vi "Diagnostics Message Loop.vi"(8 "error in (no error)":errorcluster, 11 "Message Queues":T1) -> (0 "error out":errorcluster)   [LabVIEW 2021, in "Diagnostics.lvlib"]
uses:
  Diagnostics.lvlib
  support/Message Queue/All Message Queues.ctl
  support/Message Queue/Message Cluster.ctl
  Diagnostics State.ctl
  Settings/Settings.ctl
  Acquisition/Hardware Configuration.ctl
  Acquisition/Signal Type.ctl
  Logging/Logging Configuration.ctl
  <vilib>/Utility/error.llb/Error Cluster From Error Code.vi
  <vilib>/ErrorRing/Error Ring.xnode
  Logging/Logging.lvlib
  Acquisition/Acquisition.lvlib
  Settings/Settings.lvlib
  support/Message Queue/Message Queue.lvlib
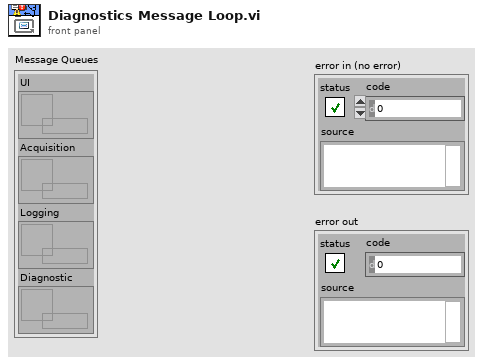
[diagram p1: front panel]
types:
  T1 = typedef "Message Queue.lvlib/All Message Queues.ctl" = cluster{"UI":refnum<queue>, "Acquisition":refnum<queue>, "Logging":refnum<queue>, "Diagnostic":refnum<queue>}
  T2 = typedef "Settings.lvlib/Settings.ctl" = cluster{"IO":T3, "Log":T5}
  T3 = typedef "Acquisition.lvlib/Hardware Configuration.ctl" = cluster{"HW Refnum <Replace Me>":string, "Signal Type <Replace Me>":T4}
  T4 = typedef "Acquisition.lvlib/Signal Type.ctl" = enum16{"Sine Wave", "Square with Noise"}
  T5 = typedef "Logging.lvlib/Logging Configuration.ctl" = cluster{"Path":path, "TDMS":refnum<k34>, "Spreadsheet":refnum<file>, "Append":bool}
  T6 = typedef "Diagnostics.lvlib/Diagnostics State.ctl" = enum16{"Idle", "Active"}
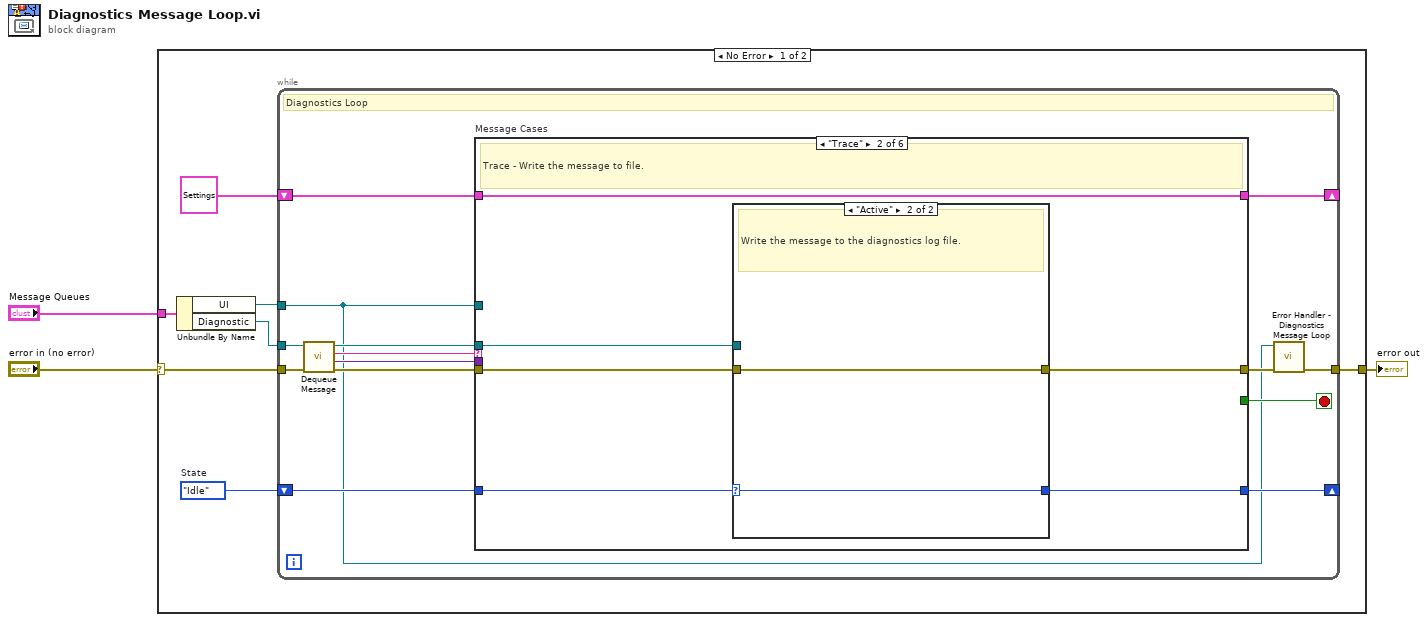
[diagram p0: block diagram]
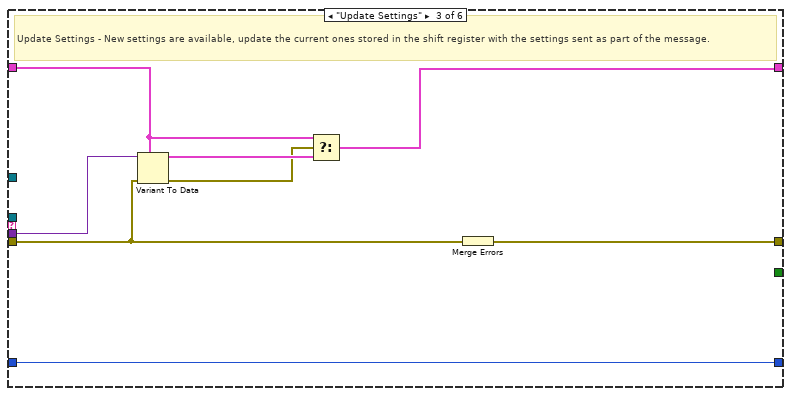
[diagram p4: hidden frame]
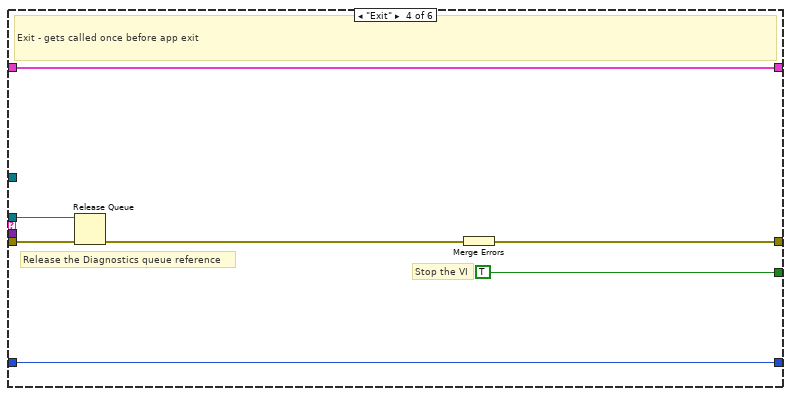
[diagram p5: hidden frame]
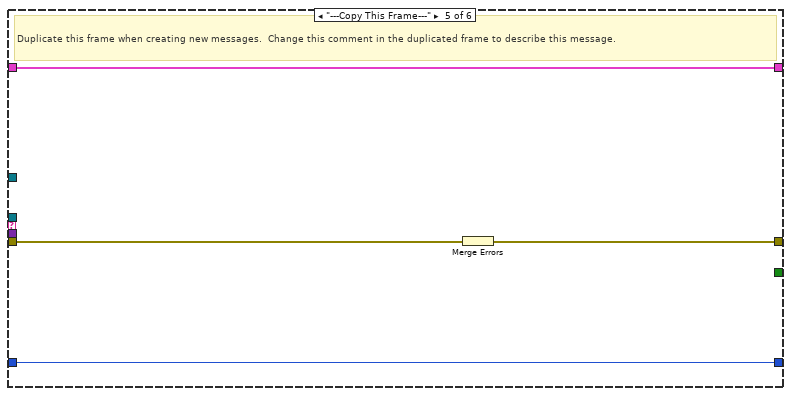
[diagram p6: hidden frame]
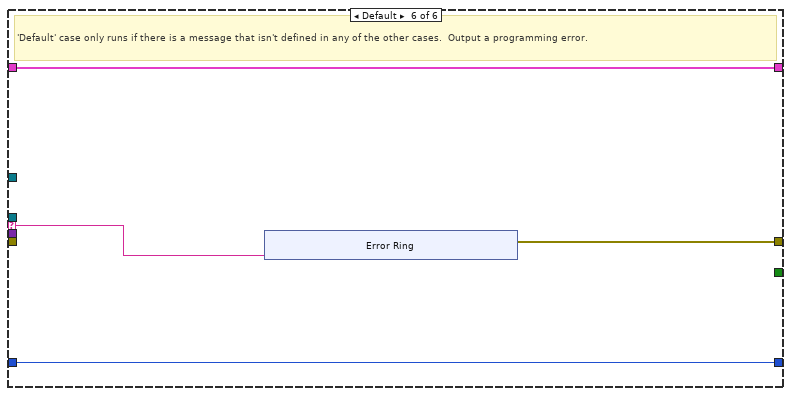
[diagram p7: hidden frame]
diagram:
  n1 = case shown="No Error" "error in (no error)" {
    selector: "error in (no error)" -> [w7 w68]
    tunnel: "Message Queues" -> [w10 _]
    tunnel: [w8 w68] -> w2
    frame No Error {
      w5 = Diagnostics_State."Idle"  # State
      n2 = Unbundle By Name(w10) -> ("UI"=w6:refnum<queue>, "Diagnostic"=w9:refnum<queue>)
      n3 = while {
        tunnel: w9 -> [w16]
        shift-right: [w23] -> _
        shift-left: T2 {"IO"={"HW Refnum <Replace Me>"="", "Signal Type <Replace Me>"=enum."Sine Wave"}, "Log"={"Path"=path "", "TDMS"=refnum, "Spreadsheet"=refnum, "Append"=FALSE}} ("Settings") -> [w24]
        tunnel: w6 -> [w11]
        shift-right: [w14] -> _
        shift-left: w5 -> [w15]
        tunnel: w7 -> [w21]
        tunnel: [w13] -> w8
        stop <- w22 stop-if-true
        # "Diagnostics Loop"
        n4 = call "Dequeue Message.vi"("error in (no error)"=w21, "Message Queue"=w16) -> ("error out"=w20:errorcluster, "Message Data"=w18:variant, "Message"=w19:string, "dup Message Queue"=w17:refnum<queue>)  [unwired: 6 in]
        n5 = case "Message Cases" shown="\"Trace\"" w19 {
          selector: w19 -> [_ _ _ _ _ w57]
          tunnel: w17 -> [_ w32 _ w49 _ _]
          tunnel: w20 -> [w26 w31 w39 w50 w56 _]
          tunnel: [w26 w33 w45 w51 w54 w58] -> w12
          tunnel: w24 -> [w27 w30 w43 w46 w55 w60]
          tunnel: [w27 w30 w40 w46 w55 w60] -> w23
          tunnel: [_ _ _ TRUE _ _] -> w22
          tunnel: w18 -> [_ _ w44 _ _ _]
          tunnel: w11 -> [_ _ _ _ _ _]
          tunnel: w15 -> [w25 w29 w38 w47 w53 w59]
          tunnel: [w25 w28 w38 w47 w53 w59] -> w14
          frame "Initialize" {
            # "Initialize - gets called once at first launch."
          }
          frame "Trace" {
            # "Trace - Write the message to file."
            n6 = case shown="\"Active\"" w29 {
              selector: w29 -> [w35 w37]
              tunnel: [w34 w36] -> w33
              tunnel: w32 -> [_ _]
              tunnel: w31 -> [w34 w36]
              tunnel: [w35 w37] -> w28
              frame "Idle" {
                # "Ignore \"Trace\" messages when idle."
              }
              frame "Active" {
                # "Write the message to the diagnostics log file."
              }
            }
          }
          frame "Update Settings" {
            # "Update Settings - New settings are available, update the current ones stored in the shift register with the settings sent as part of the message."
            n7 = Variant To Data(error in=w39, type=w43, Variant=w44) -> (data=w42:T2, error out=w41:errorcluster)
            n8 = Select(t=w43, s=w41, f=w42) -> (s? t:f=w40:T2)
            n9 = Merge Errors(w39) -> (w45:errorcluster)
          }
          frame "Exit" {
            # "Release the Diagnostics queue reference"
            # "Stop the VI"
            # "Exit - gets called once before app exit"
            n10 = Release Queue(queue=w49, error in (no error)=w50) -> (error out=w48:errorcluster)  [unwired: 1 in, 2 out]
            n11 = Merge Errors(w48) -> (w51:errorcluster)
          }
          frame "---Copy This Frame---" {
            # "Duplicate this frame when creating new messages.  Change this comment in the duplicated frame to describe this message."
            n12 = Merge Errors(w56) -> (w54:errorcluster)
          }
          frame Default {
            # "'Default' case only runs if there is a message that isn't defined in any of the other cases.  Output a programming error."
            n13 = xnode "Error Ring"("parameter 0"=w57) -> ("error out"=w58:errorcluster)
          }
        }
        n14 = call "Error Handler - Diagnostics Message Loop.vi"("error in (no error)"=w12, "Message Queue"=w11) -> ("dup error in"=w13:errorcluster)  [unwired: 8 in, 1 out]
      }
    }
    frame Error {
    }
  }
  "error out" <- w2
